vi "Close Hardware.vi"(8 "error in (no error)":errorcluster, 11 "Instrument.Oxford1820 in":refnum<class "Instrument.Oxford1820.lvclass">) -> (0 "error out":errorcluster, 3 "Instrument.Oxford1820 out":refnum<class "Instrument.Oxford1820.lvclass">)   [LabVIEW 2019, in "Instrument.Oxford1820.lvclass"]
uses:
  Instrument.Oxford1820.lvclass
  <instrlib>/Mercury iXX/Public/Controls/Mercury Reference.ctl
  <instrlib>/Mercury iXX/Public/Controls/Comms Transport Layer.ctl
  <instrlib>/Mercury iXX/Private/Controls/Query Dynamic Reference.ctl
  Instrument.Oxford1820.lvclass/Instrument.Oxford1820.ctl
  <instrlib>/Mercury iXX/Mercury iXX.lvlib
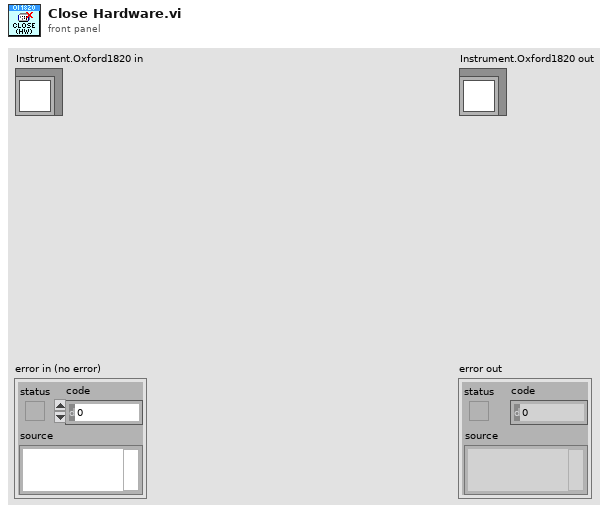
[diagram p1: front panel]
types:
  T1 = typedef "Mercury iXX.lvlib/Mercury Reference.ctl" = cluster{"Comms":refnum<visa-resource-name>, "Device ID":string[], "Comms Layer":T2, "Command":string, "Query reference":T3}
  T2 = typedef "Mercury iXX.lvlib/Comms Transport Layer.ctl" = enum16{"Ethernet TCP/IP", "USB", "ISOBus - RS-232", "GPIB"}
  T3 = typedef "Mercury iXX.lvlib/Query Dynamic Reference.ctl" = refnum<vi>
  T4 = cluster{"Reference":T1, "Devices":cluster{"Auxiliary":string, "Pressure":string, "Heater":string, "Temperature":string, "Lambda":string}}
  T5 = cluster{"Reference":T1, "Devices":cluster{"Level":string, "Temperature":string, "Magnet":string, "PSU1":string, "PSU2":string, "PSU3":string}}
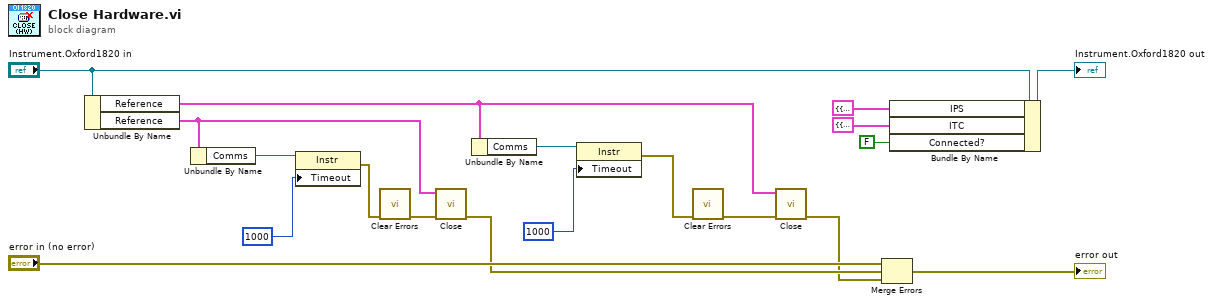
[diagram p0: block diagram]
diagram:
  n1 = Unbundle By Name("Instrument.Oxford1820 in") -> ("Reference"=w8:T1, "Reference"=w12:T1)
  n2 = Unbundle By Name(w12) -> ("Comms"=w14:refnum<visa-resource-name>)
  n3 = property class="Instr"(reference=w14, "Timeout"=u32 1000 ("General Settings:Timeout Value")) -> (error out=w11:errorcluster)  [unwired: 1 in, 1 out]
  n4 = call <vilib>:"Clear Errors.vi"("error in (no error)"=w11) -> ("error out"=w6:errorcluster)  [unwired: 5 in, 1 out]
  n5 = call <instrlib>:"Close.vi"("error in (no error)"=w6, "Mercury Reference"=w12) -> ("error out"=w3:errorcluster)  [unwired: 9 out]
  n6 = Unbundle By Name(w8) -> ("Comms"=w9:refnum<visa-resource-name>)
  n7 = property class="Instr"(reference=w9, "Timeout"=u32 1000 ("General Settings:Timeout Value")) -> (error out=w7:errorcluster)  [unwired: 1 in, 1 out]
  n8 = call <vilib>:"Clear Errors.vi"("error in (no error)"=w7) -> ("error out"=w5:errorcluster)  [unwired: 5 in, 1 out]
  n9 = call <instrlib>:"Close.vi"("error in (no error)"=w5, "Mercury Reference"=w8) -> ("error out"=w2:errorcluster)  [unwired: 9 out]
  n10 = Merge Errors("error in (no error)", w3, w2) -> (→"error out":errorcluster)
  n11 = Bundle By Name(cluster="Instrument.Oxford1820 in", "IPS"=T5 {"Reference"={"Comms"="", "Device ID"=[], "Comms Layer"=enum."Ethernet TCP/IP", "Command"="", "Query reference"=refnum}, "Devices"={"Level"="", "Temperature"="", "Magnet"="", "PSU1"="", "PSU2"="", "PSU3"=""}}, "ITC"=T4 {"Reference"={"Comms"="", "Device ID"=[], "Comms Layer"=enum."Ethernet TCP/IP", "Command"="", "Query reference"=refnum}, "Devices"={"Auxiliary"="", "Pressure"="", "Heater"="", "Temperature"="", "Lambda"=""}}, "Connected?"=FALSE ("Connection.Connected?")) -> (→"Instrument.Oxford1820 out":refnum<class "Instrument.Oxford1820.lvclass">)
